vi "svfa_Check for AvgParam Change.vi"(6 "averaging parameters":T1={"averaging mode"=enum."No averaging", "weighting mode"=enum."Linear", "number of averages"=10, "linear mode"=enum."Auto restart"}, 7 "restart averaging (F)":bool, 8 "error in (no error)":errorcluster) -> (0 "error out":errorcluster, 2 "parameter has changed":bool)   [LabVIEW 2017]
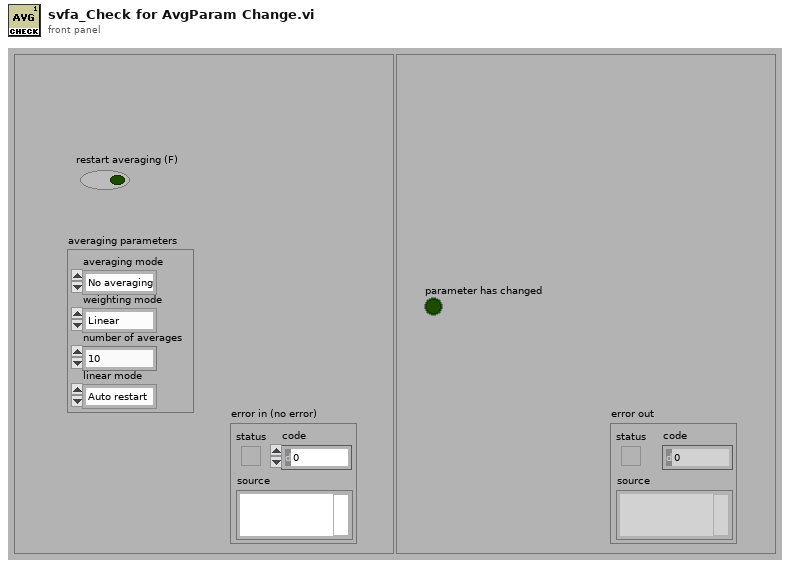
[diagram p1: front panel]
types:
  T1 = cluster{"averaging mode":enum16{"No averaging", "Vector averaging", "RMS averaging", "Peak hold"}, "weighting mode":enum16{"Linear", "Exponential"}, "number of averages":u32, "linear mode":enum16{"One shot", "Auto restart"}}
  T2 = enum16{"No averaging", "Vector averaging", "RMS averaging", "Peak hold"}
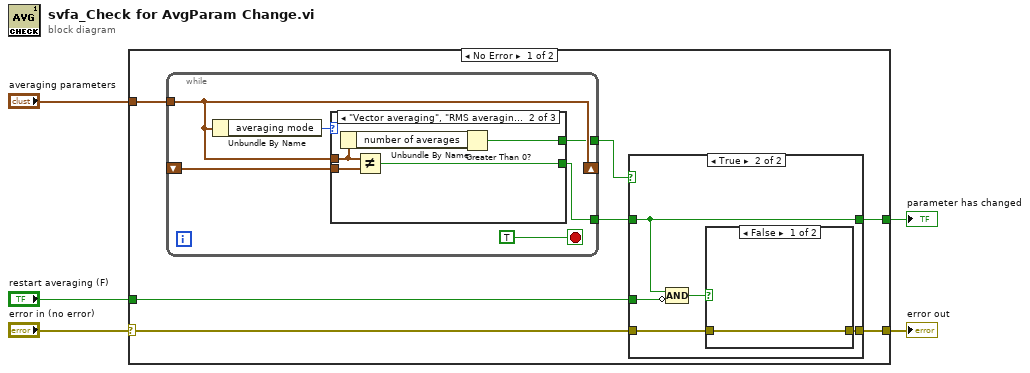
[diagram p0: block diagram]
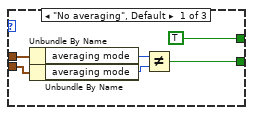
[diagram p2: hidden frame]
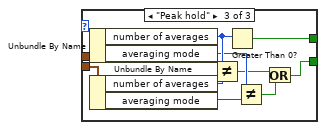
[diagram p3: hidden frame]
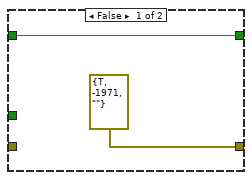
[diagram p4: hidden frame]
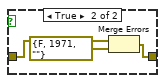
[diagram p5: hidden frame]
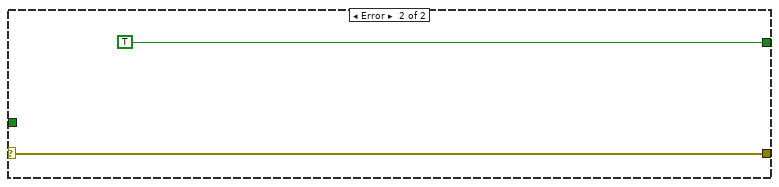
[diagram p6: hidden frame]
diagram:
  n1 = case shown="No Error" "error in (no error)" {
    selector: "error in (no error)" -> [w11 w52]
    tunnel: [w10 w52] -> w2
    tunnel: "averaging parameters" -> [w12 _]
    tunnel: [w7 TRUE] -> w3
    tunnel: "restart averaging (F)" -> [w6 _]
    frame No Error {
      n2 = while {
        tunnel: [w13] -> w8
        tunnel: [w16] -> w9
        tunnel: w12 -> [w14]
        shift-left: _ -> [w17]
        shift-right: [w14] -> _
        stop <- TRUE stop-if-true
        n3 = Unbundle By Name(w14) -> ("averaging mode"=w15:T2)
        n4 = case shown="\"Vector averaging\", \"RMS averaging\"" w15 {
          tunnel: w14 -> [w23 w28 w39]
          tunnel: w17 -> [w22 w29 w38]
          tunnel: [w21 w27 w30] -> w16
          tunnel: [TRUE w25 w37] -> w13
          frame "No averaging", Default {
            n5 = Unbundle By Name(w23) -> ("averaging mode"=w19:T2)
            n6 = Unbundle By Name(w22) -> ("averaging mode"=w20:T2)
            n7 = Not Equal?(x=w19, y=w20) -> (x != y?=w21:bool)
          }
          frame "Vector averaging", "RMS averaging" {
            n8 = Unbundle By Name(w28) -> ("number of averages"=w26:u32)
            n9 = Not Equal?(x=w28, y=w29) -> (x != y?=w27:bool)
            n10 = Greater Than 0?(x=w26) -> (x > 0?=w25:bool)
          }
          frame "Peak hold" {
            n11 = Unbundle By Name(w39) -> ("number of averages"=w36:u32, "averaging mode"=w34:T2)
            n12 = Unbundle By Name(w38) -> ("number of averages"=w35:u32, "averaging mode"=w33:T2)
            n13 = Not Equal?(x=w36, y=w35) -> (x != y?=w32:bool)
            n14 = Greater Than 0?(x=w36) -> (x > 0?=w37:bool)
            n15 = Not Equal?(x=w34, y=w33) -> (x != y?=w31:bool)
            n16 = Or(x=w32, y=w31) -> (x .or. y?=w30:bool)
          }
        }
      }
      n17 = case shown="True" w8 {
        tunnel: w11 -> [_ w46]
        tunnel: [errorcluster {"status"=TRUE, "code"=-1971, "source"=""} ("error IO") w45] -> w10
        tunnel: w9 -> [w40 w44]
        tunnel: [w40 w44] -> w7
        tunnel: w6 -> [_ w42]
        frame False {
        }
        frame True {
          n18 = Compound Arithmetic op=AND(w44, invert w42) -> (w43:bool)
          n19 = case shown="False" w43 {
            tunnel: w46 -> [w47 w50]
            tunnel: [w47 w48] -> w45
            frame False {
            }
            frame True {
              n20 = Merge Errors(w50, errorcluster {"status"=FALSE, "code"=1971, "source"=""} ("error IO")) -> (w48:errorcluster)
            }
          }
        }
      }
    }
    frame Error {
    }
  }
  "error out" <- w2
  "parameter has changed" <- w3
